vi "Demo - Change Phase Offset.vi"(9 "Phase Offset (Radians) in":dbl[](array[numeric]), 10 "Channel":i32, 11 "x":dbl) -> (1 "Phase Offset (Radians) out":dbl[](array[numeric]))   [LabVIEW 2017]
doc: "Increments the array of phase offset data."
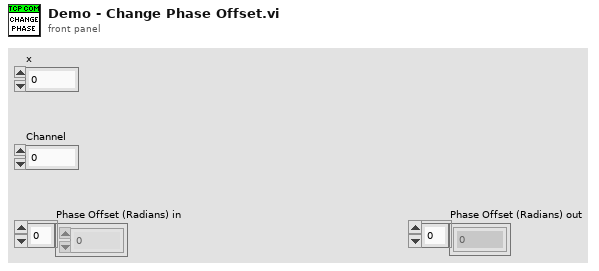
[diagram p1: front panel]
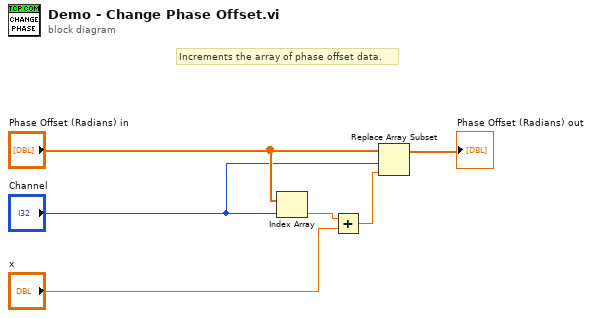
[diagram p0: block diagram]
diagram:
  # "Increments the array of phase offset data."
  n1 = Index Array(array="Phase Offset (Radians) in", index="Channel") -> (element=w4:dbl)
  n2 = Add(x=w4, y="x") -> (x+y=w2:dbl)
  n3 = Replace Array Subset(array="Phase Offset (Radians) in", new element=w2, index="Channel") -> (→"Phase Offset (Radians) out":dbl[])
